vi "ReadFormulaParameter.vi"(1 "reference":refnum<vi>) -> (0 "FormulaParameter":T4)   [LabVIEW 2013]
uses:
  <vilib>/Utility/miscctls.llb/LVBoundsTypeDef.ctl
  <vilib>/Utility/miscctls.llb/LVPositionTypeDef.ctl
  <vilib>/Utility/miscctls.llb/LVRectTypeDef.ctl
panel:
  out "error out 17":errorcluster
  out "error out 16":errorcluster
  out "error out 15":errorcluster
  out "error out 14":errorcluster
  out "error out 13":errorcluster
  out "error out 12":errorcluster
  out "error out 11":errorcluster
  out "error out 10":errorcluster
  out "error out 9":errorcluster
  out "error out 8":errorcluster
  out "error out 7":errorcluster
  out "error out 6":errorcluster
  out "error out 5":errorcluster
  out "error out 4":errorcluster
  out "error out 3":errorcluster
  out "error out 2":errorcluster
  out "error out":errorcluster
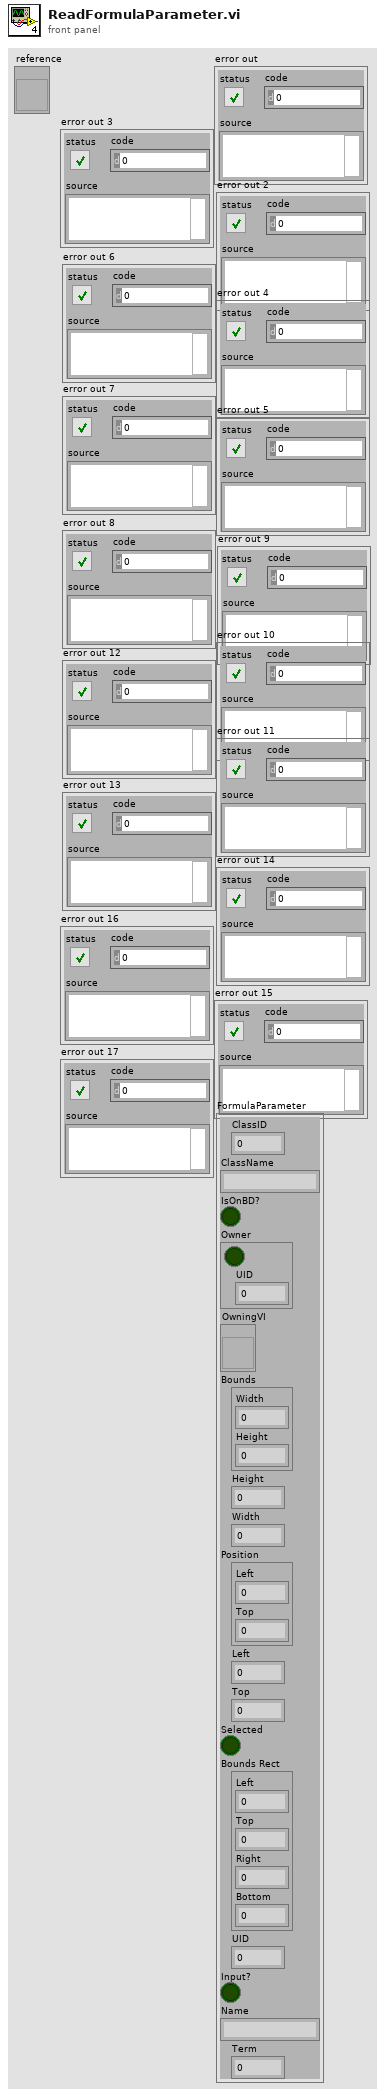
[diagram p1: front panel]
types:
  T1 = typedef "LVBoundsTypeDef.ctl" = cluster{"Width":u32, "Height":u32}
  T2 = typedef "LVPositionTypeDef.ctl" = cluster{"Left":i32, "Top":i32}
  T3 = typedef "LVRectTypeDef.ctl" = cluster{"Left":i16, "Top":i16, "Right":i16, "Bottom":i16}
  T4 = cluster{"ClassID":u32, "ClassName":string, "IsOnBD?":bool, "Owner":cluster{bool, "UID":i32}, "OwningVI":refnum<vi>, "Bounds":T1, "Height":u32, "Width":u32, "Position":T2, "Left":i32, "Top":i32, "Selected":bool, "Bounds Rect":T3, "UID":i32, "Input?":bool, "Name":string, "Term":i32}
  T5 = cluster{"ClassID":u32, "ClassName":string, "IsOnBD?":bool, "Cluster":cluster{bool, "UID":i32}, "OwningVI":refnum<vi>, "Bounds":T1, "Height":u32, "Width":u32, "Position":T2, "Left":i32, "Top":i32, "Selected":bool, "Bounds Rect":T3, "UID":i32, "Input?":bool, "Name":string, "UID":i32}
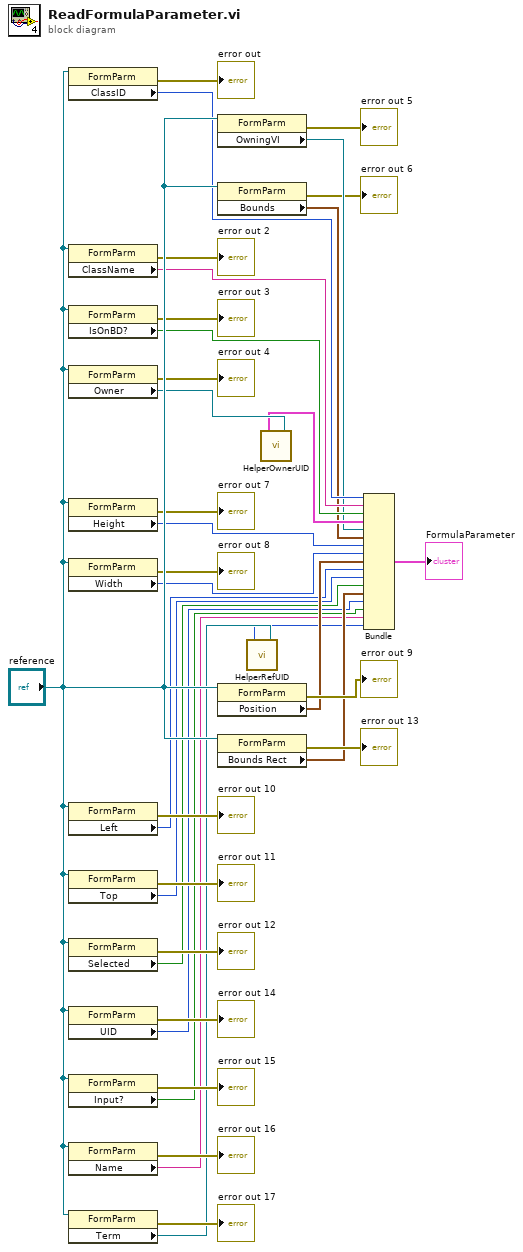
[diagram p0: block diagram]
diagram:
  n1 = property class="FormParm"(reference="reference") -> (error out=→"error out":errorcluster, "ClassID"=w36:u32)  [unwired: 1 in, 1 out]
  n2 = property class="FormParm"(reference="reference") -> (error out=→"error out 2":errorcluster, "ClassName"=w34:string)  [unwired: 1 in, 1 out]
  n3 = property class="FormParm"(reference="reference") -> (error out=→"error out 3":errorcluster, "IsOnBD?"=w32:bool)  [unwired: 1 in, 1 out]
  n4 = property class="FormParm"(reference="reference") -> (error out=→"error out 4":errorcluster, "Owner"=w30:refnum<vi>)  [unwired: 1 in, 1 out]
  n5 = property class="FormParm"(reference="reference") -> (error out=→"error out 7":errorcluster, "Height"=w23:u32)  [unwired: 1 in, 1 out]
  n6 = property class="FormParm"(reference="reference") -> (error out=→"error out 8":errorcluster, "Width"=w21:u32)  [unwired: 1 in, 1 out]
  n7 = property class="FormParm"(reference="reference") -> (error out=→"error out 10":errorcluster, "Left"=w17:i32)  [unwired: 1 in, 1 out]
  n8 = property class="FormParm"(reference="reference") -> (error out=→"error out 11":errorcluster, "Top"=w15:i32)  [unwired: 1 in, 1 out]
  n9 = property class="FormParm"(reference="reference") -> (error out=→"error out 12":errorcluster, "Selected"=w13:bool)  [unwired: 1 in, 1 out]
  n10 = property class="FormParm"(reference="reference") -> (error out=→"error out 14":errorcluster, "UID"=w9:i32)  [unwired: 1 in, 1 out]
  n11 = property class="FormParm"(reference="reference") -> (error out=→"error out 15":errorcluster, "Input?"=w7:bool)  [unwired: 1 in, 1 out]
  n12 = property class="FormParm"(reference="reference") -> (error out=→"error out 16":errorcluster, "Name"=w5:string)  [unwired: 1 in, 1 out]
  n13 = property class="FormParm"(reference="reference") -> (error out=→"error out 17":errorcluster, "Term"=w3:refnum<vi>)  [unwired: 1 in, 1 out]
  n14 = property class="FormParm"(reference="reference") -> (error out=→"error out 5":errorcluster, "OwningVI"=w27:refnum<vi>)  [unwired: 1 in, 1 out]
  n15 = property class="FormParm"(reference="reference") -> (error out=→"error out 6":errorcluster, "Bounds"=w25:T1)  [unwired: 1 in, 1 out]
  n16 = property class="FormParm"(reference="reference") -> (error out=→"error out 9":errorcluster, "Position"=w19:T2)  [unwired: 1 in, 1 out]
  n17 = property class="FormParm"(reference="reference") -> (error out=→"error out 13":errorcluster, "Bounds Rect"=w11:T3)  [unwired: 1 in, 1 out]
  n18 = call "HelperRefUID.vi"("Text in"=w3) -> ("UID"=w2:i32)
  n19 = call "HelperOwnerUID.vi"("Generic in"=w30) -> ("Cluster"=w29:cluster{bool, "UID":i32})
  n20 = Bundle("ClassID"=w36, "ClassName"=w34, "IsOnBD?"=w32, "Cluster"=w29, "OwningVI"=w27, "Bounds"=w25, "Height"=w23, "Width"=w21, "Position"=w19, "Left"=w17, "Top"=w15, "Selected"=w13, "Bounds Rect"=w11, "UID"=w9, "Input?"=w7, "Name"=w5, "UID"=w2) -> (→"FormulaParameter":T5)  [unwired: 1 in]
